vi "Format to string.vi"(8 "error in (no error)":errorcluster, 11 "address":refnum<class "Hostname Network Address.lvclass">) -> (0 "error out":errorcluster, 2 "String":string, 3 "address out":refnum<class "Hostname Network Address.lvclass">)   [LabVIEW 2020, in "NI_WFCN.lvlib" / "Hostname Network Address.lvclass"]
doc: "Returns a human-readable string representation of this address."
uses:
  <vilib>/net/WFCN/Addressing/Hostname Network Address/Hostname Network Address.lvclass
  <vilib>/net/WFCN/Addressing/Hostname Network Address/Hostname Network Address.lvclass/Hostname Network Address.ctl
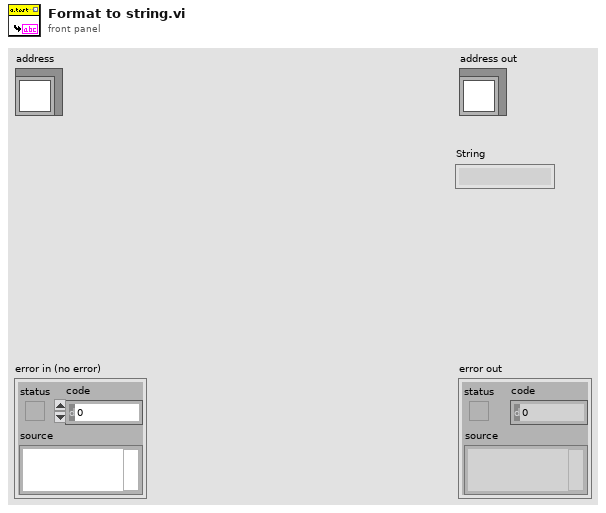
[diagram p1: front panel]
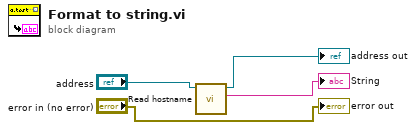
[diagram p0: block diagram]
diagram:
  n1 = call <vilib>:"Read hostname.vi"("address"="address") -> ("hostname"=→"String":string, "address out"=→"address out":refnum<class "Hostname Network Address.lvclass">)  [unwired: 9 in]
  "error out" <- "error in (no error)"
